vi "LoadDashboardServer.vi"(0 "Universal Robot in":refnum<class "Universal Robot.lvclass">, 1 "DashboardServer":refnum<class "Dashboard Server.lvclass">, 5 "error in (no error)":errorcluster) -> (14 "Universal Robot out":refnum<class "Universal Robot.lvclass">, 19 "error out":errorcluster)   [LabVIEW 2019, in "Universal Robot.lvclass"]
uses:
  Universal Robot.lvclass
  Client Interfaces/Dashboard Server/Dashboard Server.lvclass
  Universal Robot.lvclass/Universal Robot.ctl
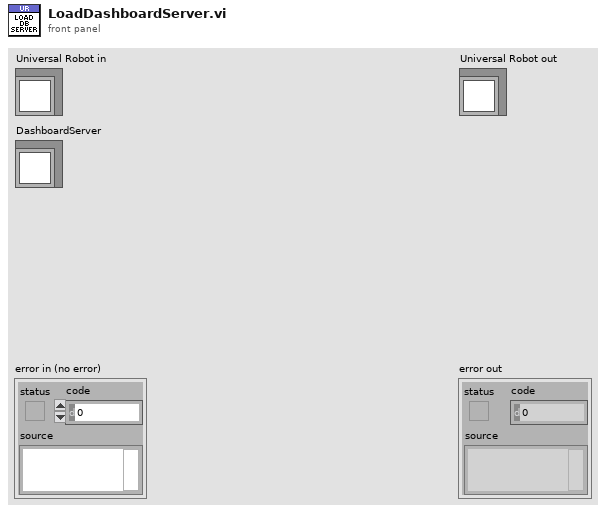
[diagram p1: front panel]
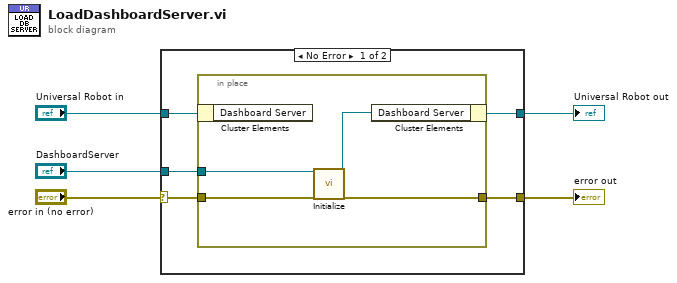
[diagram p0: block diagram]
diagram:
  n1 = case shown="No Error" "error in (no error)" {
    selector: "error in (no error)" -> [w10 w16]
    tunnel: [w8 w16] -> w4
    tunnel: [w6 w15] -> w2
    tunnel: "Universal Robot in" -> [w7 w15]
    tunnel: "DashboardServer" -> [w9 _]
    frame No Error {
      n2 = in-place {
        in-place-border: w10 -> [w14]
        in-place-border: w9 -> [w13]
        in-place-border: [w12] -> w8
        n3 = in-place-cluster #1(w7) -> ()  [unwired: 1 out]
        n4 = call-dynamic "Initialize.vi"("DashboardServer in"=w13, "error in (no error)"=w14) -> ("DashboardServer out"=w11:refnum<class "Dashboard Server.lvclass">, "error out"=w12:errorcluster)  [unwired: 16 in]
        n5 = in-place-cluster #1("Dashboard Server"=w11) -> (w6:refnum<class "Universal Robot.lvclass">)
      }
    }
    frame Error {
    }
  }
  "error out" <- w4
  "Universal Robot out" <- w2
